vi "Close.vi"(8 "error in (no error)":errorcluster, 11 "Data in":refnum<class "Alias Bus.lvclass">) -> (0 "error out":errorcluster, 3 "Data out":refnum<class "Alias Bus.lvclass">)   [LabVIEW 2021, in "Alias Bus.lvclass"]
doc: "Abstract Data Classes 2.1.1.12\nTim Streeter - TSA\nCopyright (c) 2024, TSA"
uses:
  Alias Bus.lvclass
  Alias Bus.lvclass/Alias Bus.ctl
  Properties/Read Buses.vi
  Omni-Bus/Bus Access/Bus_Access.lvclass
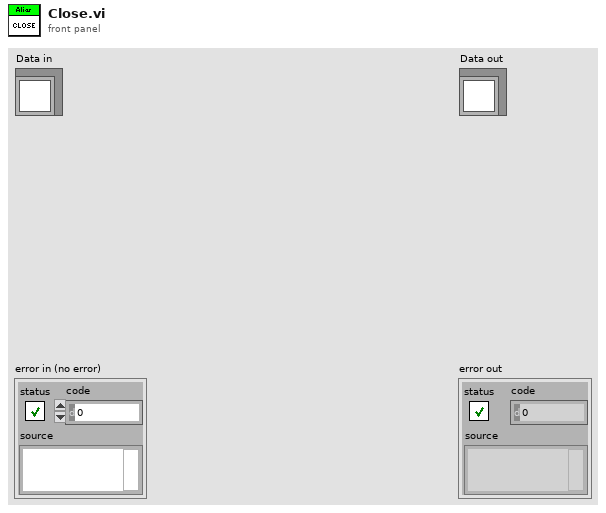
[diagram p1: front panel]
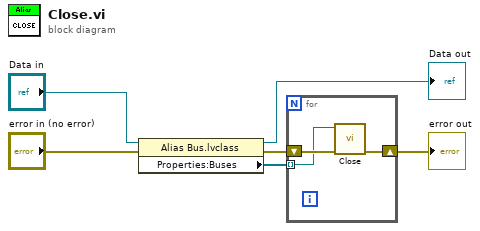
[diagram p0: block diagram]
diagram:
  n1 = property class="Alias Bus.lvclass"(reference="Data in", error in="error in (no error)") -> (reference out=→"Data out":refnum<class "Alias Bus.lvclass">, error out=w4:errorcluster, "Properties:Buses"=w3:refnum<class "Bus_Access.lvclass">[])
  n2 = for {
    tunnel: w3 -> [w8] mode=indexing
    shift-right: [w7] -> w1
    shift-left: w4 -> [w9]
    n3 = call-dynamic "Close.vi"("error in (no error)"=w9, "Data in"=w8) -> ("error out"=w7:errorcluster)  [unwired: 8 in, 1 out]
  }
  "error out" <- w1
